vi "Read JSON Type.vi"(8 "error in (no error)":errorcluster, 11 "Variant in":variant) -> (0 "error out":errorcluster, 2 "datatype":T1, 3 "JSON Value out":variant)   [LabVIEW 2020, in "Variant JSON API.lvlib"]
doc: "Returns the JSON Type of the given object. This may be used to determine if the value of a control of type JSON Null, JSON Literal or JSON Structured Type is an instance of a more specific type."
uses:
  Variant JSON API.lvlib
  JSON Type.ctl
  Errors.ctl
  <vilib>/Utility/Data Type/NI_Data Type.lvlib
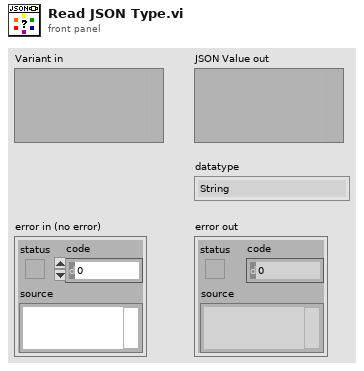
[diagram p1: front panel]
types:
  T1 = typedef "Variant JSON API.lvlib/JSON Type.ctl" = enum16{"String", "Numeric", "Boolean", "NULL", "Object", "Array"}
  T2 = typedef "Variant JSON API.lvlib/Errors.ctl" = enum16{"No key", "Key path type", "Array OOB", "Type Mismatch", "Invalid Token", "Invalid Value"}
  T3 = typedef "NI_Data Type.lvlib/Data Type.ctl" = enum8{"Invalid Type", "Void", "I8", "I16", "I32", "I64", "U8", "U16", "U32", "U64", "Single Float", "Double Float", "Extended Float", "Single Complex", "Double Complex", "Extended Complex", "Enum U8", "Enum U16", "Enum U32", "Enum U64", "Single Float With Unit", "Double Float With Unit", "Extended Float With Unit", "Single Complex with Unit", "Double Complex with Unit", "Extended Complex with Unit", "Boolean", "String", "Path", "Picture", "Tag", "Array", "Cluster", "Variant", "LV Variant", "Waveform", "Timestamp", "Digital Waveform", "Digital Data", "ExpressData", "Refnum", "External Data", "VI", "Poly VI", "LabVIEW Class Instance", "Fixed Point", "Set Collection", "Map Collection"}
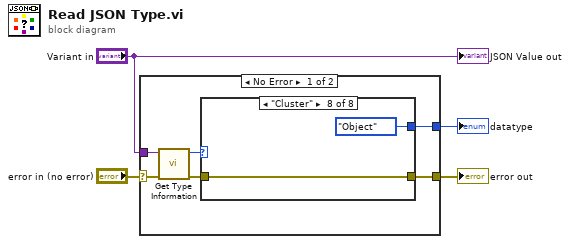
[diagram p0: block diagram]
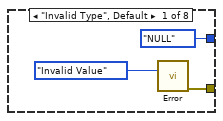
[diagram p2: hidden frame]
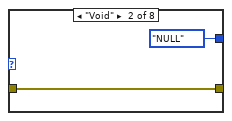
[diagram p3: hidden frame]
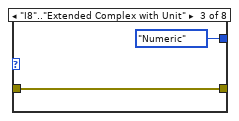
[diagram p4: hidden frame]
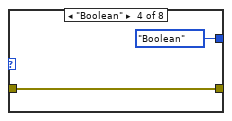
[diagram p5: hidden frame]
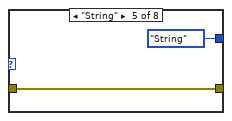
[diagram p6: hidden frame]
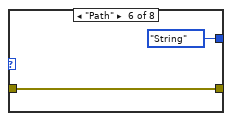
[diagram p7: hidden frame]
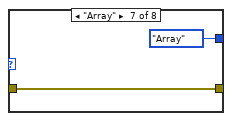
[diagram p8: hidden frame]
diagram:
  n1 = case shown="No Error" "error in (no error)" {
    selector: "error in (no error)" -> [w9 w28]
    tunnel: "Variant in" -> [w10 _]
    tunnel: [w7 _] -> w2
    tunnel: [w5 w28] -> w1
    frame No Error {
      n2 = call <vilib>:"Get Type Information.vi"("error in (no error)"=w9, "variant"=w10) -> ("error out"=w6:errorcluster, "type"=w8:T3)  [unwired: 5 in, 3 out]
      n3 = case shown="\"Cluster\"" w8 {
        tunnel: [JSON_Type."NULL" ("datatype") JSON_Type."NULL" ("datatype") JSON_Type."Numeric" ("datatype") JSON_Type."Boolean" ("datatype") JSON_Type."String" ("datatype") JSON_Type."String" ("datatype") JSON_Type."Array" ("datatype") JSON_Type."Object" ("datatype")] -> w7
        tunnel: w6 -> [_ w14 w16 w18 w20 w22 w24 w26]
        tunnel: [w11 w14 w16 w18 w20 w22 w24 w26] -> w5
        frame "Invalid Type", Default {
          n4 = call "Error.vi"(5:Errors."Invalid Value") -> ("error out"=w11:errorcluster)  [unwired: 14 in]
        }
        frame "Void" {
        }
        frame "I8".."Extended Complex with Unit" {
        }
        frame "Boolean" {
        }
        frame "String" {
        }
        frame "Path" {
        }
        frame "Array" {
        }
        frame "Cluster" {
        }
      }
    }
    frame Error {
    }
  }
  "error out" <- w1
  "datatype" <- w2
  "JSON Value out" <- "Variant in"
